vi "CENTRIOD DETECTION BEAMPOINTING.vi"(0 "Refnum in":T7=refnum, 4 "beam detection para":T5={"Filter"=1, "Filter Para"={"X Size"=5, "Y Size"=5, "% Tolerance"=1}, "detection method"=4, "smal para"=[{"Measurement Parameter"=35, "Range Lower Value"=0.0, "Range Upper Value"=500.0, "Range"=TRUE, "Measurement Type"=FALSE}], "Remove small Objects"=TRUE, "Restrict to round Objects"=TRUE} {"smal para"."Measurement Parameter" items=["Center of Mass X", "Center of Mass Y", "First Pixel X", "First Pixel Y", "Bounding Rect Left", "Bounding Rect Top", "Bounding Rect Right", "Bounding Rect Bottom", "Max Feret Diameter Start X", "Max Feret Diameter Start Y", "Max Feret Diameter End X", "Max Feret Diameter End Y", "Max Horiz. Segment Length Left", "Max Horiz. Segment Length Right", "Max Horiz. Segment Length Row", "-", "Bounding Rect Width", "Bounding Rect Height", "Bounding Rect Diagonal", "Perimeter", "Convex Hull Perimeter", "Holes' Perimeter", "Max Feret Diameter", "Equivalent Ellipse Major Axis", "Equivalent Ellipse Minor Axis", "Equivalent Ellipse Minor Axis (Feret)", "Equivalent Rect Long Side", "Equivalent Rect Short Side", "Equivalent Rect Diagonal", "Equivalent Rect Short Side (Feret)", "Average Horiz. Segment Length", "Average Vert. Segment Length", "Hydraulic Radius", "Waddel Disk Diameter", "-", "Area", "Holes' Area", "Particle & Holes' Area", "Convex Hull Area", "Image Area", "-", "Number of Holes", "Number of Horiz. Segments", "Number of Vert. Segments", "-", "Orientation", "Max Feret Diameter Orientation", "-", "% Area/Image Area", "% Area/(Particle & Holes' Area)", "Ratio of Equivalent Ellipse Axes", "Ratio of Equivalent Rect Sides", "-", "Elongation Factor", "Compactness Factor", "Heywood Circularity Factor", "Type Factor", "-", "Sum X", "Sum Y", "Sum XX", "Sum XY", "Sum YY", "Sum XXX", "Sum XXY", "Sum XYY", "Sum YYY", "-", "Moment of Inertia XX", "Moment of Inertia XY", "Moment of Inertia YY", "Moment of Inertia XXX", "Moment of Inertia XXY", "Moment of Inertia XYY", "Moment of Inertia YYY", "Norm. Moment of Inertia XX", "Norm. Moment of Inertia XY", "Norm. Moment of Inertia YY", "Norm. Moment of Inertia XXX", "Norm. Moment of Inertia XXY", "Norm. Moment of Inertia XYY", "Norm. Moment of Inertia YYY", "Hu Moment 1", "Hu Moment 2", "Hu Moment 3", "Hu Moment 4", "Hu Moment 5", "Hu Moment 6", "Hu Moment 7"]; "smal para"."Range Lower Value" format="%.2f"; "smal para"."Range Upper Value" format="%.2f"; "detection method" items=["clustering", "entropy", "metric", "moments", "inter-class variance"]; "Filter" items=["No Filter", "Median Filter", "Low Pass Filter"]}, 5 "error in (no error)":errorcluster) -> (8 "Bounding Rect":T8={"Left"=200.0, "Top"=222.0, "Right"=337.0, "Bottom"=354.0}, 11 "Particle Reports (Pixels)":T9(array[cluster])=[{"Area"=13217.0, "Number of Holes"=0.0, "Bounding Rect"={"Left"=200.0, "Top"=222.0, "Right"=337.0, "Bottom"=354.0}, "Center of Mass"={"X"=269.13989558901415, "Y"=287.03949459030036}, "Orientation"=28.32814462161336, "Dimensions"={"Width"=137.0, "Height"=132.0}}] {"Orientation" format="%.2f"; "Dimensions"."Height" format="%.2f"; "Dimensions"."Width" format="%.2f"; "Center of Mass"."Y" format="%.2f"; "Center of Mass"."X" format="%.2f"; "Bounding Rect"."Bottom" format="%.2f"; "Bounding Rect"."Right" format="%.2f"; "Bounding Rect"."Top" format="%.2f"; "Bounding Rect"."Left" format="%.2f"; "Number of Holes" format="%.2f"; "Area" format="%.2f"}, 13 "Area":dbl=13217.0, 14 "Refnum out":T7, 17 "Number of Particles":i32=1, 18 "Centriod":cluster{"X":dbl, "Y":dbl}={"X"=268.53924560546875, "Y"=286.7691955566406}, 19 "error out":errorcluster)   [LabVIEW 2020]
uses:
  <vilib>/vision/Image Controls.llb/IMAQ Image.ctl
  Ctrs/beam detection.ctl
  <vilib>/vision/Measure.llb/Edge Options.ctl
  <vilib>/vision/Measure.llb/Edge Polarity.ctl
  <vilib>/vision/NI_Vision_Development_Module.lvlib
panel:
  in  "Conversion Policy (Full Dynamic)":T1 {"Conversion Method" items=["Full Dynamic", "Downshift", "Given Range", "90 % Dynamic", "Given Percent Range"]}
  out "Circle Found":bool=TRUE
  in  "Options":T4={"Search  Direction"=1, "Edge Options"={"Edge Polarity"=2, "Kernel Size"=3, "Width"=3, "Minimum Edge Strength"=10.0, "Interpolation Type"=enum."Bilinear Fixed", "Data Processing Method"=enum."Average"}, "Show Search Area"=FALSE, "Show Search Lines"=FALSE, "Show Edges Found"=FALSE, "Show Result"=TRUE, "Search Area Color"=65280, "Search Lines Color"=255, "Edge Locations Color"=16776960, "Result Color"=3079978, "Overlay Group Name"=""} {"Search  Direction" items=["Outside to Inside", "Inside to Outside"]; "Edge Options"."Edge Polarity" items=["All Edges", "Rising Edges", "Falling Edges"]; "Edge Options"."Minimum Edge Strength" format="%.2f"; "Edge Options"."Width" step=2; "Edge Options"."Kernel Size" step=2}
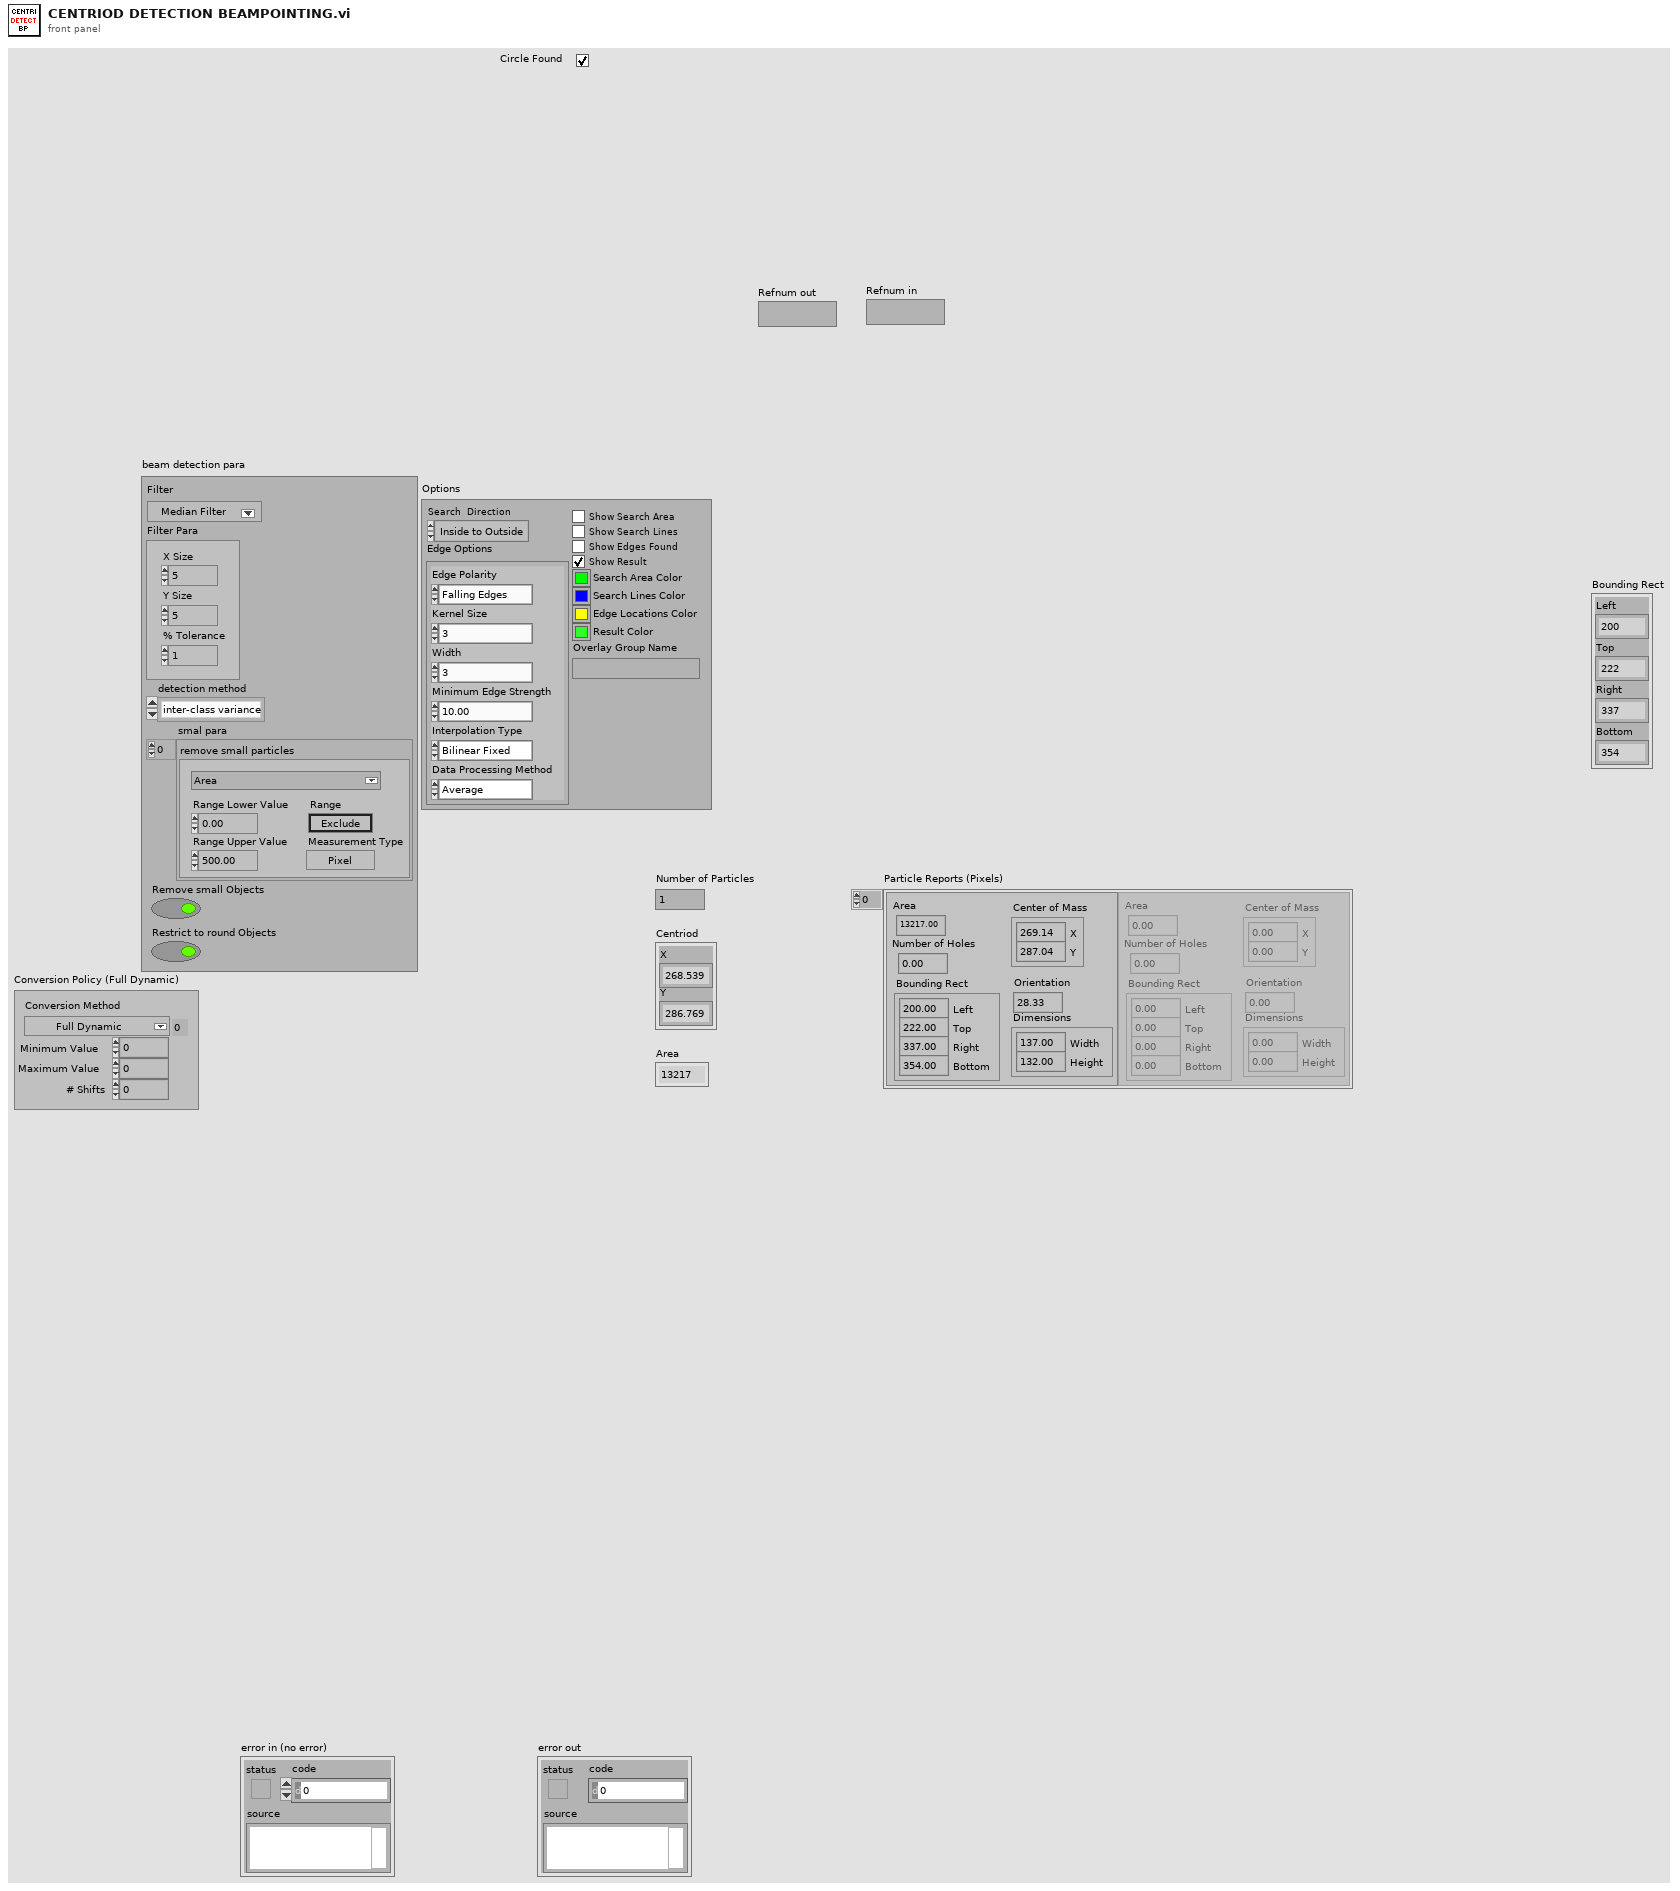
[diagram p1: front panel]
types:
  T1 = cluster{"Conversion Method":u32, "Minimum Value":i32, "Maximum Value":i32, "# Shifts":i32}
  T2 = typedef "Edge Options.ctl" = cluster{"Edge Polarity":T3, "Kernel Size":u32, "Width":u32, "Minimum Edge Strength":sgl, "Interpolation Type":enum32{"Zero Order", "Bilinear", "Quadratic", "Cubic", "Bilinear Fixed"}, "Data Processing Method":enum32{"Average", "Median"}}
  T3 = typedef "Edge Polarity.ctl" = u32
  T4 = cluster{"Search  Direction":u32, "Edge Options":T2, "Show Search Area":bool, "Show Search Lines":bool, "Show Edges Found":bool, "Show Result":bool, "Search Area Color":u32, "Search Lines Color":u32, "Edge Locations Color":u32, "Result Color":u32, "Overlay Group Name":string}
  T5 = typedef "beam detection.ctl" = cluster{"Filter":u16, "Filter Para":cluster{"X Size":i32, "Y Size":i32, "% Tolerance":i32}, "detection method":i32, "smal para":cluster{"Measurement Parameter":T6, "Range Lower Value":dbl, "Range Upper Value":dbl, "Range":bool, "Measurement Type":bool}[], "Remove small Objects":bool, "Restrict to round Objects":bool}
  T6 = typedef "Particle Parameters" = i32
  T7 = typedef "IMAQ Image.ctl" = refnum<image>
  T8 = cluster{"Left":dbl, "Top":dbl, "Right":dbl, "Bottom":dbl}
  T9 = cluster{"Area":dbl, "Number of Holes":dbl, "Bounding Rect":cluster{"Left":dbl, "Top":dbl, "Right":dbl, "Bottom":dbl}, "Center of Mass":cluster{"X":dbl, "Y":dbl}, "Orientation":dbl, "Dimensions":cluster{"Width":dbl, "Height":dbl}}[]
  T10 = typedef "Image Type" = u32
  T11 = cluster{"X Size":i32, "Y Size":i32, "% Tolerance":i32}
  T12 = typedef "IMAQ Circle" = cluster{"Center X":i32, "Center Y":i32, "Inner Radius":i32, "Outer Radius":i32, "Start Angle":dbl, "End Angle":dbl}
  T13 = cluster{"Measurement Parameter":T6, "Range Lower Value":dbl, "Range Upper Value":dbl, "Range":bool, "Measurement Type":bool}[]
  T14 = cluster{"Area":dbl, "Number of Holes":dbl, "Bounding Rect":cluster{"Left":dbl, "Top":dbl, "Right":dbl, "Bottom":dbl}, "Center of Mass":cluster{"X":dbl, "Y":dbl}, "Orientation":dbl, "Dimensions":cluster{"Width":dbl, "Height":dbl}}
  T15 = typedef "ROI Descriptor" = cluster{"Global Rectangle":i32[], "Contours":cluster{"ID":enum32{"External", "Internal"}, "Type":u32, "Coordinates":i32[]}[]}
  T16 = cluster{"Center (Pixels)":cluster{"X":sgl, "Y":sgl}, "Radius (Pixels)":dbl, "Center (Real-World)":cluster{"X":sgl, "Y":sgl}, "Radius (Real-World)":dbl, "Roundness (Real-World)":dbl, "Average Strength":dbl, "Average SNR (dB)":dbl}
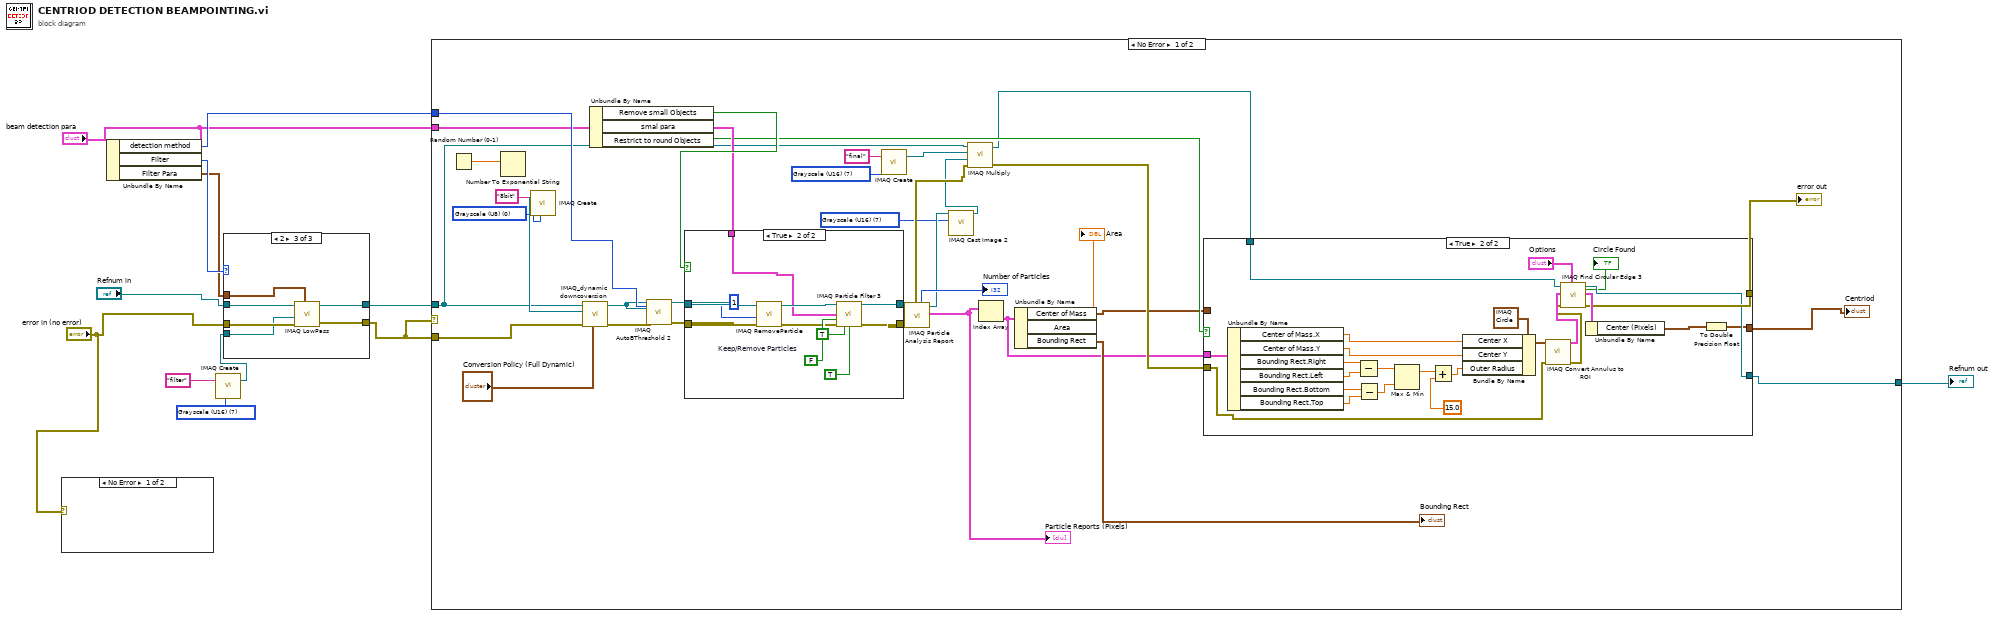
[diagram p0: block diagram]
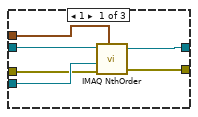
[diagram p6: hidden frame]
diagram:
  w12 = T10 7 items=["Grayscale (U8)", "Grayscale (I16)", "Grayscale (SGL)", "Complex (CSG)", "RGB (U32)", "HSL (U32)", "RGB (U64)", "Grayscale (U16)"] ("Image Type")
  n1 = case shown="No Error" "error in (no error)" {
    frame No Error {
    }
    frame Error {
    }
  }
  n2 = Unbundle By Name("beam detection para") -> ("detection method"=w9:i32, "Filter"=w10:u16, "Filter Para"=w8:T11)
  n3 = call "IMAQ Create"("Image Name"="filter", "Image Type"=w12) -> ("New Image"=w11:T7)  [unwired: 3 in, 1 out]
  n4 = case shown="2" w10 {
    tunnel: "error in (no error)" -> [w15 w19 w26]
    tunnel: "Refnum in" -> [w17 w20 w25]
    tunnel: w8 -> [w18 _ w24]
    tunnel: [w13 w20 w23] -> w1
    tunnel: w11 -> [w16 _ w22]
    tunnel: [w14 w19 w21] -> w3
    frame 1 {
      n5 = call "IMAQ NthOrder"("Image Src"=w17, "Size & Order #"=w18, "Image Dst"=w16, "error in (no error)"=w15) -> ("Image Dst Out"=w13:T7, "error out"=w14:errorcluster)  [unwired: 3 in]
    }
    frame 0, Default {
    }
    frame 2 {
      n6 = call "IMAQ LowPass"("Image Src"=w25, "Size & Tolerance"=w24, "Image Dst"=w22, "error in (no error)"=w26) -> ("Image Dst Out"=w23:T7, "error out"=w21:errorcluster)  [unwired: 3 in]
    }
  }
  n7 = case shown="No Error" w3 {
    tunnel: w3 -> [w60 _]
    tunnel: w9 -> [w51 _]
    tunnel: "beam detection para" -> [w50 _]
    tunnel: w1 -> [w32 w104]
    tunnel: [w36 w104] -> w5
    frame No Error {
      w29 = T10 7 items=["Grayscale (U8)", "Grayscale (I16)", "Grayscale (SGL)", "Complex (CSG)", "RGB (U32)", "HSL (U32)", "RGB (U64)", "Grayscale (U16)"] ("Image Type")
      w58 = T10 0 items=["Grayscale (U8)", "Grayscale (I16)", "Grayscale (SGL)", "Complex (CSG)", "RGB (U32)", "HSL (U32)", "RGB (U64)", "Grayscale (U16)"] ("Image Type")
      w56 = T10 7 items=["Grayscale (U8)", "Grayscale (I16)", "Grayscale (SGL)", "Complex (CSG)", "RGB (U32)", "HSL (U32)", "RGB (U64)", "Grayscale (U16)"] ("Image Type")
      n8 = Random Number (0-1)() -> (number: 0 to 1=w47:dbl)
      n9 = Number To Exponential String(number=w47) -> ()  [unwired: 3 in, 1 out]
      n10 = call "IMAQ Create"("Image Name"="8bit", "Image Type"=w58) -> ("New Image"=w59:T7)  [unwired: 3 in, 1 out]
      n11 = call "IMAQ_dynamic downcoversion.vi"("Conversion Policy (Full Dynamic)"="Conversion Policy (Full Dynamic)", "error in (no error)"=w60, "Image Dst"=w59, "Image Src"=w32) -> ("error out"=w27:errorcluster, "Image Out"=w35:T7)  [unwired: 6 in]
      n12 = Unbundle By Name(w50) -> ("Remove small Objects"=w49:bool, "smal para"=w48:T13, "Restrict to round Objects"=w45:bool)
      n13 = call "IMAQ AutoBThreshold 2"("Image Src"=w35, "Method (clustering)"=w51, "Image Dst"=w35, "error in (no error)"=w27) -> ("Image Dst Out"=w33:T7, "error out"=w53:errorcluster)  [unwired: 9 in, 1 out]
      n14 = case shown="True" w49 {
        tunnel: [w92 w99] -> w54
        tunnel: [w91 w98] -> w55
        tunnel: w33 -> [w92 w97]
        tunnel: w53 -> [w91 w96]
        tunnel: w48 -> [_ w94]
        frame False {
        }
        frame True {
          w103 = FALSE  # Keep/Remove Particles
          n15 = call "IMAQ RemoveParticle"("error in (no error)"=w96, "Number of Erosion"=1 ("Numeric"), "Image Src"=w97) -> ("error out"=w100:errorcluster, "Image Dst Out"=w101:T7)  [unwired: 4 in, 3 out]
          n16 = call "IMAQ Particle Filter 3"("Image Src"=w101, "Selection Values"=w94, "Keep/Remove Particles (F)"=w103, "error in (no error)"=w100, "Reject Border? (F)"=TRUE, "Fill Holes? (F)"=TRUE) -> ("Image Dst Out"=w99:T7, "error out"=w98:errorcluster)  [unwired: 3 in, 5 out]
        }
      }
      n17 = call "IMAQ Create"("Image Name"="final", "Image Type"=w56) -> ("New Image"=w57:T7)  [unwired: 3 in, 1 out]
      n18 = call "IMAQ Particle Analysis Report"("error in (no error)"=w55, "Image"=w54) -> ("error out"=w61:errorcluster, "Particle Reports (Pixels)"=w40:T9, "Image Out (duplicate)"=w30:T7, "Number of Particles"=→"Number of Particles":i32)  [unwired: 4 in, 2 out]
      "Particle Reports (Pixels)" <- w40
      n19 = call "IMAQ Cast Image 2"("Image Src"=w30, "Image Type"=w29) -> ("Image Dst Out"=w28:T7)  [unwired: 12 in, 1 out]
      n20 = call "IMAQ Multiply"("Image Src A"=w32, "Image Dst"=w57, "Image Src B"=w28, "error in (no error)"=w61) -> ("Image Dst Out"=w31:T7, "error out"=w44:errorcluster)  [unwired: 3 in]
      n21 = Index Array(array=w40) -> (element=w39:T14)  [unwired: 1 in]
      n22 = Unbundle By Name(w39) -> ("Center of Mass"=w38:cluster{"X":dbl, "Y":dbl}, "Area"=→"Area":dbl, "Bounding Rect"=→"Bounding Rect":T8)
      n23 = case shown="True" w45 {
        tunnel: w31 -> [w63 w90]
        tunnel: [w65 w83] -> w37
        tunnel: w38 -> [w65 _]
        tunnel: w44 -> [w64 w77]
        tunnel: [w64 w87] -> w43
        tunnel: [w63 w86] -> w36
        tunnel: w39 -> [_ w80]
        frame False {
        }
        frame True {
          n24 = Unbundle By Name(w80) -> ("Center of Mass.X"=w67:dbl, "Center of Mass.Y"=w66:dbl, "Bounding Rect.Right"=w72:dbl, "Bounding Rect.Left"=w71:dbl, "Bounding Rect.Bottom"=w70:dbl, "Bounding Rect.Top"=w69:dbl)
          n25 = Subtract(x=w72, y=w71) -> (x-y=w73:dbl)
          n26 = Subtract(x=w70, y=w69) -> (x-y=w74:dbl)
          n27 = Max & Min(x=w73, y=w74) -> (max(x,y)=w75:dbl)  [unwired: 1 out]
          n28 = Add(x=w75, y=15.0) -> (x+y=w68:dbl)
          n29 = Bundle By Name(cluster=T12 {"Center X"=0, "Center Y"=0, "Inner Radius"=0, "Outer Radius"=0, "Start Angle"=0.0, "End Angle"=360.0} ("Annulus"), "Center X"=w67, "Center Y"=w66, "Outer Radius"=w68) -> (w81:T12)
          n30 = call "IMAQ Convert Annulus to ROI"("error in (no error)"=w77, "Annulus"=w81) -> ("error out"=w78:errorcluster, "ROI Descriptor"=w79:T15)  [unwired: 7 in]
          n31 = call "IMAQ Find Circular Edge 3"("Options"="Options", "error in (no error)"=w78, "ROI Descriptor"=w79, "Image"=w90) -> ("error out"=w87:errorcluster, "Fitted Circle"=w88:T16, "Image Out"=w86:T7, "Circle Found"=→"Circle Found":bool)  [unwired: 3 in, 1 out]
          n32 = Unbundle By Name(w88) -> ("Center (Pixels)"=w84:cluster{"X":sgl, "Y":sgl})
          n33 = To Double Precision Float(number=w84) -> (double precision float=w83:cluster{"X":dbl, "Y":dbl})
        }
      }
      "error out" <- w43
      "Centriod" <- w37
    }
    frame Error {
    }
  }
  "Refnum out" <- w5
